vi "Robot Global Data.vi"() -> ()   [LabVIEW 2017]
doc: "This global VI can contain as many global variables as you need. To create a global variable, place a control on the panel, give it a good name. To read or write to it from a VI, drag the icon to the diagram of that VI. You can also drag from the project. Click on the node to change which global you access. You shouldn't have multiple locations writing to a global or it will cause a race-condition."
uses:
  <vilib>/Rock Robotics/WPI/Camera/WPI_CameraImageSize.ctl
  <vilib>/Rock Robotics/WPI/DriverStation/WPI_DriverStationRobotMode2.ctl
  2018_Trobots_5013_Dashboard/Routines and Block Data.ctl
  Support Code/Blocks.ctl
panel:
  in  "Routines and Block Data":T1
  in  "Gyro Refnum Ready":bool
  in  "Robot Mode":T3
  in  "image size":T4=enum."320x240"
  in  "Enable Vision":bool
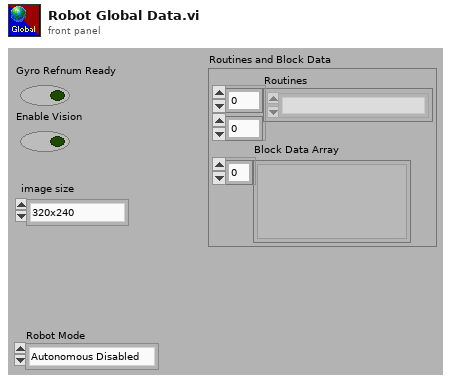
[diagram p1: front panel]
types:
  T1 = typedef "Routines and Block Data.ctl" = cluster{"Routines":T2[][], "Block Data Array":variant[]}
  T2 = typedef "Blocks.ctl" = enum16{"", "Wait 1s", "Far to L1", "L1 to End Switch 1", "End Switch 1 to Corridor", "End Cube to C1", "C1 to Diag Scale 1", "C1 to C3", "C3 to C4", "Diag Scale to C1", "C3 to End Switch 2", "C3 to Cube&Switch", "Middle to Front S2", "Middle to Front S1", "Front S1 to Line 1", "Front S2 to Line 2", "End Switch 1 to End Cube", "Line 1 to C1"}
  T3 = typedef "WPI_DriverStationRobotMode2.ctl" = enum16{"Autonomous Disabled", "Autonomous Enabled", "Teleop Disabled", "Teleop Enabled", "Disconnected", "Finish", "Test Disabled", "Test Enabled", "Emergency Stopped"}
  T4 = typedef "WPI_CameraImageSize.ctl" = enum16{"640x480", "320x240", "160x120", "Custom"}
diagram:
